vi "controlSensorDirection.vi"(7 "Set":bool, 8 "error in":errorcluster, 9 "Inverted":bool, 10 "axis in":u8, 11 "connection ID":refnum<k5>) -> (0 "error out":errorcluster, 1 "Inverted":bool, 2 "axis out":i32, 3 "connection ID":refnum<k5>)   [LabVIEW 2016]
doc: "This function retrieves or sets the IDS sensor source of closed loop to inverted when true."
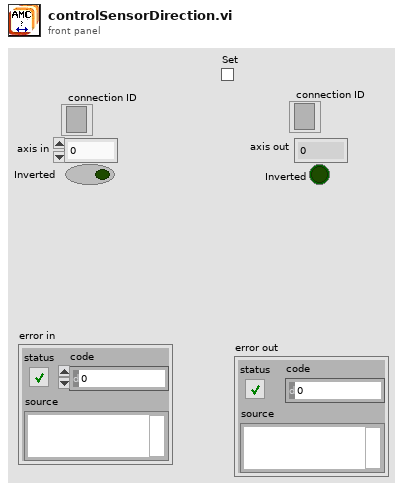
[diagram p1: front panel]
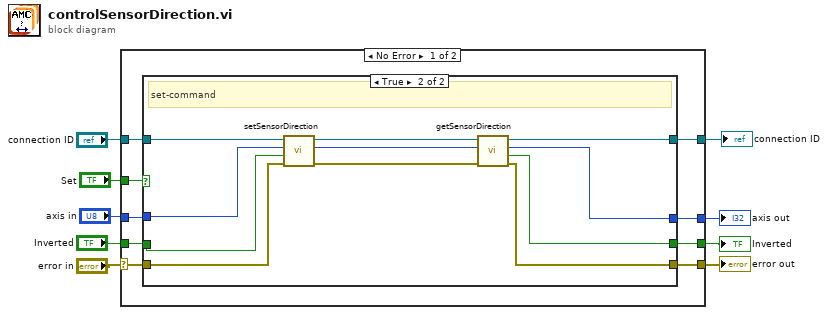
[diagram p0: block diagram]
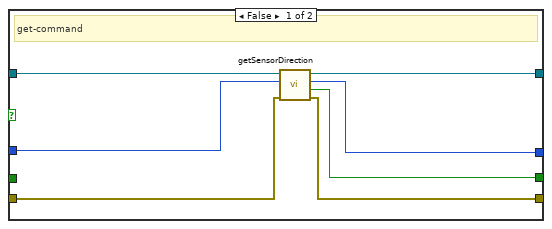
[diagram p2: hidden frame]
diagram:
  n1 = case shown="No Error" "error in" {
    selector: "error in" -> [w14 w40]
    tunnel: "axis in" -> [w18 w37]
    tunnel: [w11 w40] -> w8
    tunnel: "Inverted" -> [w16 w38]
    tunnel: [w13 w38] -> w3
    tunnel: "Set" -> [w15 _]
    tunnel: [w12 w39] -> w6
    tunnel: "connection ID" -> [w17 w39]
    tunnel: [w10 w37] -> w1
    frame No Error {
      n2 = case shown="True" w15 {
        tunnel: w17 -> [w25 w36]
        tunnel: w18 -> [w23 w35]
        tunnel: w16 -> [_ w34]
        tunnel: w14 -> [w22 w27]
        tunnel: [w19 w29] -> w13
        tunnel: [w24 w30] -> w12
        tunnel: [w21 w32] -> w11
        tunnel: [w20 w26] -> w10
        frame False {
          # "get-command"
          n3 = call "getSensorDirection.vi"("error in"=w22, "axis"=w23, "connection ID"=w25) -> ("error out"=w21:errorcluster, "inverted"=w19:bool, "axis_out"=w20:i32, "connection ID"=w24:refnum<k5>)  [unwired: 5 in]
        }
        frame True {
          # "set-command"
          n4 = call "setSensorDirection.vi"("error in"=w27, "inverted"=w34, "axis"=w35, "connection ID"=w36) -> ("error out"=w33:errorcluster, "axis_out"=w28:i32, "connection ID"=w31:refnum<k5>)  [unwired: 5 in]
          n5 = call "getSensorDirection.vi"("error in"=w33, "axis"=w28, "connection ID"=w31) -> ("error out"=w32:errorcluster, "inverted"=w29:bool, "axis_out"=w26:i32, "connection ID"=w30:refnum<k5>)  [unwired: 5 in]
        }
      }
    }
    frame Error {
    }
  }
  "error out" <- w8
  "axis out" <- w1
  "Inverted" <- w3
  "connection ID" <- w6
